vi "ConfigureAdvancedSequencerElement.vi"(4 "error in (no error)":errorcluster, 5 "Sequencer Element":i16=1, 6 "Advanced Sequencer Item":T1={"Entry Length"=16384, "Repetition Count"=1, "Infinite Repetitions"=FALSE, "Channels"=[{"Analog Waveform"="SINE", "Amplitude [V]"=2.0, "Offset [V]"=0.0}, {"Analog Waveform"="SINE", "Amplitude [V]"=2.0, "Offset [V]"=0.0}], "Digital Waveform"="", "Wait Event"=0, "Jump Event"=0, "Jump To Mode"=2, "Jump To Entry Item (N)"=1, "Go To Mode"=2, "Go To Entry Item (N)"=1, "Pattern Mode"=2, "Pattern Code"=1, "Pattern Jump To Entry Item (N)"=1, "Pattern Event"=0} {"Pattern Event" items=["Pattern", "Ext.Mod."]; "Pattern Jump To Entry Item (N)" min=1; "Pattern Code" min=1; "Pattern Mode" items=["First", "Previous", "Next", "Last", "Item"]; "Go To Entry Item (N)" min=1; "Go To Mode" items=["First", "Previous", "Next", "Last", "Item"]; "Jump To Entry Item (N)" min=1; "Jump To Mode" items=["First", "Previous", "Next", "Last", "Item"]; "Jump Event" items=["None", "Button", "Timer", "External", "Ext.Mod."]; "Wait Event" items=["None", "Button", "Timer", "External", "Ext.Mod."]; "Repetition Count" min=1}, 7 "VISA resource name":refnum<visa-resource-name>) -> (0 "error out":errorcluster, 3 "VISA resource name out":refnum<visa-resource-name>)   [LabVIEW 2020, in "Active Technologies AWG3000.lvlib"]
uses:
  Active Technologies AWG3000.lvlib
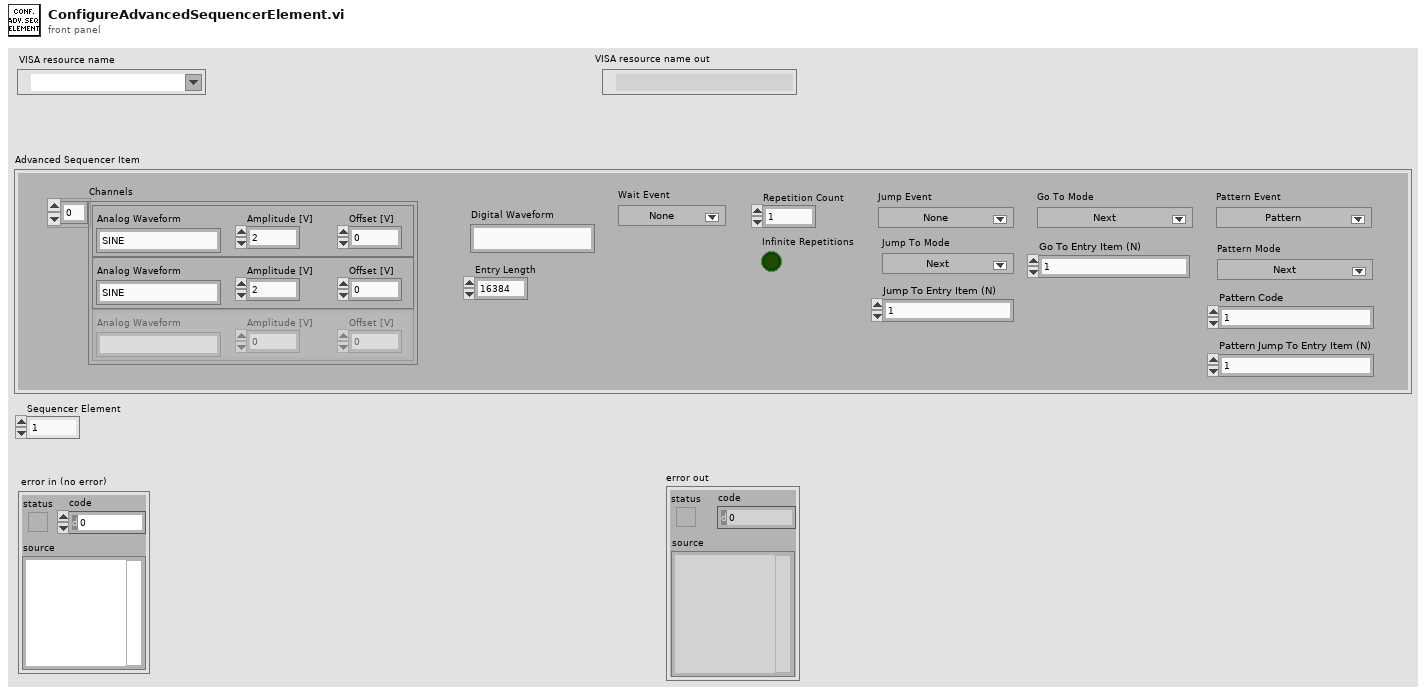
[diagram p1: front panel]
types:
  T1 = cluster{"Entry Length":i32, "Repetition Count":i32, "Infinite Repetitions":bool, "Channels":cluster{"Analog Waveform":string, "Amplitude [V]":dbl, "Offset [V]":dbl}[], "Digital Waveform":string, "Wait Event":u16, "Jump Event":u16, "Jump To Mode":u16, "Jump To Entry Item (N)":i32, "Go To Mode":u16, "Go To Entry Item (N)":i32, "Pattern Mode":u16, "Pattern Code":u8, "Pattern Jump To Entry Item (N)":i32, "Pattern Event":u16}
  T2 = cluster{"Analog Waveform":string, "Amplitude [V]":dbl, "Offset [V]":dbl}[]
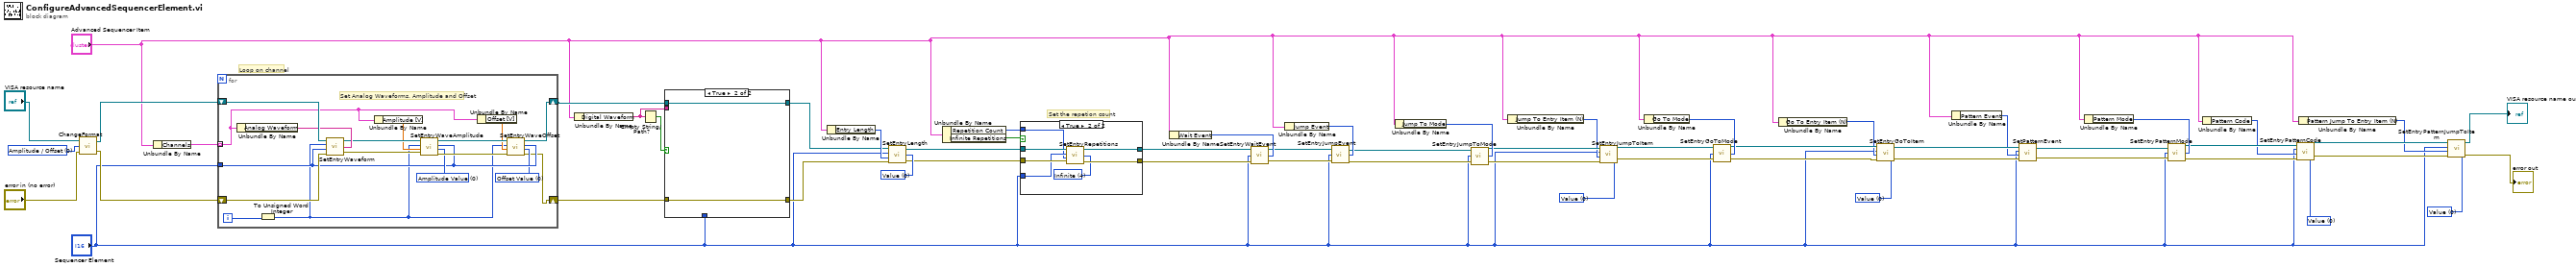
[diagram p0: block diagram]
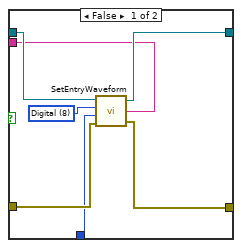
[diagram p2: hidden frame]
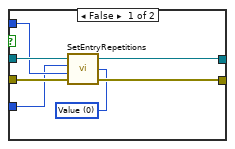
[diagram p3: hidden frame]
diagram:
  w11 = u16 0 items=["Value", "Default", "Minimum", "Maximum"] ("Jump To Entry Item Options")
  w14 = u16 0 items=["Value", "Default", "Minimum", "Maximum"] ("Pattern Code Options")
  w20 = u16 0 items=["Value", "Default", "Minimum", "Maximum"] ("Go To Entry Item Options")
  w26 = u16 0 items=["Value", "Default", "Minimum", "Maximum"] ("Jump To Entry Item Options")
  w45 = u8 0 items=["Amplitude / Offset", "Voltage High / Voltage Low"] ("Format")
  w54 = u16 0 items=["Value", "Default", "Minimum", "Maximum"] ("Entry Length Options")
  # "Set the repetion count"
  # "Loop on channel"
  n1 = call "ChangeFormat.vi"("error in (no error)"="error in (no error)", "Format"=w45, "VISA resource name"="VISA resource name") -> ("error out"=w46:errorcluster, "VISA resource name out"=w48:refnum<visa-resource-name>)
  n2 = Unbundle By Name("Advanced Sequencer Item") -> ("Channels"=w56:T2)
  n3 = for {
    tunnel: w56 -> [w60] mode=indexing
    tunnel: "Sequencer Element" -> [w63]
    shift-right: [w59] -> w42
    shift-left: w48 -> [w73]
    shift-right: [w58] -> w41
    shift-left: w46 -> [w72]
    i -> [w61]
    w62 = u16 0 items=["Offset Value", "Default", "Minimum", "Maximum"] ("Offset Options")
    w65 = u16 0 items=["Amplitude Value", "Default", "Minimum", "Maximum"] ("Amplitude Options")
    # "Set Analog Waveforms, Amplitude and Offset"
    n4 = Unbundle By Name(w60) -> ("Analog Waveform"=w71:string)
    n5 = To Unsigned Word Integer(number=w61) -> (unsigned 16bit integer=w57:u16)
    n6 = call "SetEntryWaveform.vi"("Waveform Name"=w71, "error in (no error)"=w72, "Element"=w63, "Channel"=w57, "VISA resource name"=w73) -> ("error out"=w69:errorcluster, "VISA resource name out"=w70:refnum<visa-resource-name>)
    n7 = Unbundle By Name(w60) -> ("Amplitude [V]"=w68:dbl)
    n8 = call "SetEntryWaveAmplitude.vi"("Amplitude Options"=w65, "Element"=w63, "error in (no error)"=w69, "Amplitude (Vpp)"=w68, "Channel"=w57, "VISA resource name"=w70) -> ("error out"=w66:errorcluster, "VISA resource name out"=w67:refnum<visa-resource-name>)
    n9 = Unbundle By Name(w60) -> ("Offset [V]"=w64:dbl)
    n10 = call "SetEntryWaveOffset.vi"("Offset Options"=w62, "Element"=w63, "error in (no error)"=w66, "Offset (V)"=w64, "Channel"=w57, "VISA resource name"=w67) -> ("error out"=w58:errorcluster, "VISA resource name out"=w59:refnum<visa-resource-name>)
  }
  n11 = Unbundle By Name("Advanced Sequencer Item") -> ("Digital Waveform"=w43:string)
  n12 = Empty String/Path?(string/path=w43) -> (empty?=w44:bool)
  n13 = case shown="True" w44 {
    tunnel: w42 -> [w80 w82]
    tunnel: [w79 w82] -> w40
    tunnel: [w77 w81] -> w39
    tunnel: w41 -> [w78 w81]
    tunnel: "Sequencer Element" -> [w76 _]
    tunnel: w43 -> [w75 _]
    frame False {
      w74 = u16 8 items=["Channel 1", "Channel 2", "Channel 3", "Channel 4", "Channel 5", "Channel 6", "Channel 7", "Channel 8", "Digital"] ("Channel")
      n14 = call "SetEntryWaveform.vi"("Waveform Name"=w75, "error in (no error)"=w78, "Element"=w76, "Channel"=w74, "VISA resource name"=w80) -> ("error out"=w77:errorcluster, "VISA resource name out"=w79:refnum<visa-resource-name>)
    }
    frame True {
    }
  }
  n15 = Unbundle By Name("Advanced Sequencer Item") -> ("Entry Length"=w55:i32)
  n16 = call "SetEntryLength.vi"("Entry Length Options"=w54, "error in (no error)"=w39, "Length (N)"=w55, "Element"="Sequencer Element", "VISA resource name"=w40) -> ("error out"=w52:errorcluster, "VISA resource name out"=w53:refnum<visa-resource-name>)
  n17 = Unbundle By Name("Advanced Sequencer Item") -> ("Repetition Count"=w50:i32, "Infinite Repetitions"=w51:bool)
  n18 = case shown="True" w51 {
    tunnel: w53 -> [w89 w96]
    tunnel: w52 -> [w88 w95]
    tunnel: w50 -> [w87 w90]
    tunnel: [w86 w94] -> w38
    tunnel: [w85 w93] -> w36
    tunnel: "Sequencer Element" -> [w84 w91]
    frame False {
      w83 = u16 0 items=["Value", "Default", "Minimum", "Maximum"] ("Entry Repetitions Options")
      n19 = call "SetEntryRepetitions.vi"("Entry Repetitions Options"=w83, "error in (no error)"=w88, "Entry Repetitions (N)"=w87, "Element"=w84, "VISA resource name"=w89) -> ("error out"=w85:errorcluster, "VISA resource name out"=w86:refnum<visa-resource-name>)
    }
    frame True {
      w92 = u16 4 items=["Value", "Default", "Minimum", "Maximum", "Infinite"] ("Entry Repetitions Options")
      n20 = call "SetEntryRepetitions.vi"("Entry Repetitions Options"=w92, "error in (no error)"=w95, "Entry Repetitions (N)"=w90, "Element"=w91, "VISA resource name"=w96) -> ("error out"=w93:errorcluster, "VISA resource name out"=w94:refnum<visa-resource-name>)
    }
  }
  n21 = Unbundle By Name("Advanced Sequencer Item") -> ("Wait Event"=w37:u16)
  n22 = call "SetEntryWaitEvent.vi"("Wait Event"=w37, "error in (no error)"=w36, "Element"="Sequencer Element", "VISA resource name"=w38) -> ("error out"=w34:errorcluster, "VISA resource name out"=w35:refnum<visa-resource-name>)
  n23 = Unbundle By Name("Advanced Sequencer Item") -> ("Jump Event"=w33:u16)
  n24 = call "SetEntryJumpEvent.vi"("Jump Event"=w33, "error in (no error)"=w34, "Element"="Sequencer Element", "VISA resource name"=w35) -> ("error out"=w31:errorcluster, "VISA resource name out"=w32:refnum<visa-resource-name>)
  n25 = Unbundle By Name("Advanced Sequencer Item") -> ("Jump To Mode"=w30:u16)
  n26 = call "SetEntryJumpToMode.vi"("Jump To Mode"=w30, "error in (no error)"=w31, "Element"="Sequencer Element", "VISA resource name"=w32) -> ("error out"=w28:errorcluster, "VISA resource name out"=w29:refnum<visa-resource-name>)
  n27 = Unbundle By Name("Advanced Sequencer Item") -> ("Jump To Entry Item (N)"=w27:i32)
  n28 = call "SetEntryJumpToItem.vi"("Jump To Entry Item Options"=w26, "error in (no error)"=w28, "Jump To Entry Item (N)"=w27, "Element"="Sequencer Element", "VISA resource name"=w29) -> ("error out"=w23:errorcluster, "VISA resource name out"=w24:refnum<visa-resource-name>)
  n29 = Unbundle By Name("Advanced Sequencer Item") -> ("Go To Mode"=w25:u16)
  n30 = call "SetEntryGoToMode.vi"("Go To Mode"=w25, "error in (no error)"=w23, "Element"="Sequencer Element", "VISA resource name"=w24) -> ("error out"=w21:errorcluster, "VISA resource name out"=w22:refnum<visa-resource-name>)
  n31 = Unbundle By Name("Advanced Sequencer Item") -> ("Go To Entry Item (N)"=w19:i32)
  n32 = call "SetEntryGoToItem.vi"("Go To Entry Item Options"=w20, "error in (no error)"=w21, "Go To Entry Item (N)"=w19, "Element"="Sequencer Element", "VISA resource name"=w22) -> ("error out"=w6:errorcluster, "VISA resource name out"=w7:refnum<visa-resource-name>)
  n33 = Unbundle By Name("Advanced Sequencer Item") -> ("Pattern Event"=w2:u16)
  n34 = call "SetPatternEvent.vi"("error in (no error)"=w6, "Pattern Event"=w2, "Element"="Sequencer Element", "VISA resource name"=w7) -> ("error out"=w4:errorcluster, "VISA resource name out"=w5:refnum<visa-resource-name>)
  n35 = Unbundle By Name("Advanced Sequencer Item") -> ("Pattern Mode"=w18:u16)
  n36 = call "SetEntryPatternMode.vi"("Pattern Mode"=w18, "error in (no error)"=w4, "Element"="Sequencer Element", "VISA resource name"=w5) -> ("error out"=w16:errorcluster, "VISA resource name out"=w17:refnum<visa-resource-name>)
  n37 = Unbundle By Name("Advanced Sequencer Item") -> ("Pattern Code"=w15:u8)
  n38 = call "SetEntryPatternCode.vi"("Pattern Code Options"=w14, "error in (no error)"=w16, "Pattern Code"=w15, "Element"="Sequencer Element", "VISA resource name"=w17) -> ("error out"=w12:errorcluster, "VISA resource name out"=w13:refnum<visa-resource-name>)
  n39 = Unbundle By Name("Advanced Sequencer Item") -> ("Pattern Jump To Entry Item (N)"=w10:i32)
  n40 = call "SetEntryPatternJumpToItem.vi"("Jump To Entry Item Options"=w11, "error in (no error)"=w12, "Pattern Jump To Entry Item (N)"=w10, "Element"="Sequencer Element", "VISA resource name"=w13) -> ("error out"=→"error out":errorcluster, "VISA resource name out"=→"VISA resource name out":refnum<visa-resource-name>)
